vi "SetSetpoint1.vi"(8 "Error In":errorcluster, 10 "Setpoint (C)":dbl, 11 "Omega CSi32 In":refnum<visa-resource-name>) -> (0 "Error Out":errorcluster, 3 "Omega CSi32 Out":refnum<visa-resource-name>)   [LabVIEW 2012, in "Omega-CSi32.lvlib"]
uses:
  Omega-CSi32.lvlib
panel:
  out "read buffer":string
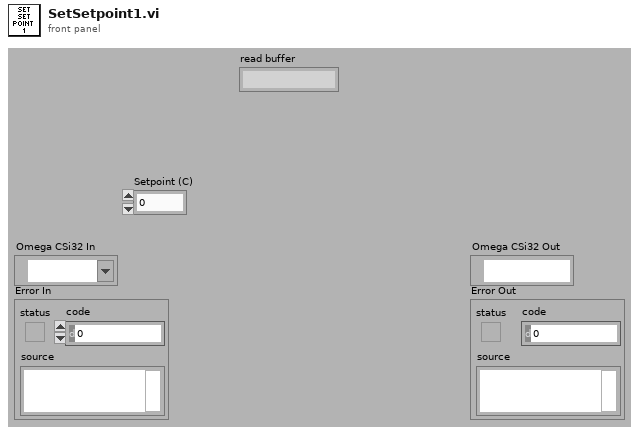
[diagram p1: front panel]
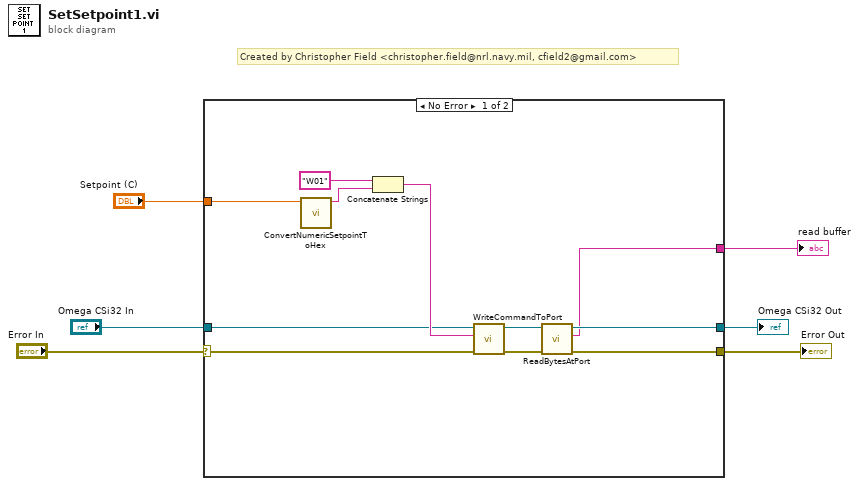
[diagram p0: block diagram]
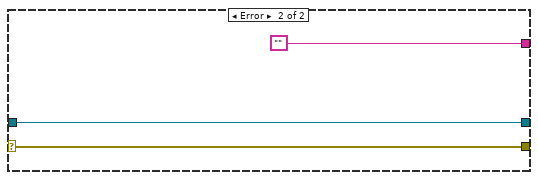
[diagram p2: hidden frame]
diagram:
  # "Created by Christopher Field <christopher.field@nrl.navy.mil, cfield2@gmail.com>"
  n1 = case shown="No Error" "Error In" {
    selector: "Error In" -> [w7 w19]
    tunnel: "Setpoint (C)" -> [w17 _]
    tunnel: "Omega CSi32 In" -> [w13 w20]
    tunnel: [w10 w20] -> w4
    tunnel: [w9 w19] -> w3
    tunnel: [w8 ""] -> w2
    frame No Error {
      n2 = call "ConvertNumericSetpointToHex.vi"("Numeric Setpoint (C)"=w17) -> ("Hex Setpoint (C)"=w16:string)  [unwired: 10 in]
      n3 = Concatenate Strings("W01" ("Command"), w16) -> (w14:string)
      n4 = call "WriteCommandToPort.vi"("Error In"=w7, "Command"=w14, "CSi32 In"=w13) -> ("Error Out"=w11:errorcluster, "CSi32 Out"=w12:refnum<visa-resource-name>)  [unwired: 7 in]
      n5 = call "ReadBytesAtPort.vi"("Error In"=w11, "CSi32 In"=w12) -> ("Error Out"=w9:errorcluster, "Read Buffer"=w8:string, "CSi32 Out"=w10:refnum<visa-resource-name>)  [unwired: 7 in]
    }
    frame Error {
    }
  }
  "Omega CSi32 Out" <- w4
  "Error Out" <- w3
  "read buffer" <- w2
